vi "AlliGator Select Phasor Plot ROI.vi"(8 "Error In":errorcluster, 11 "ROI Selection Data":cluster{"Action":T1, "ROI ID":i32}) -> (0 "Error Out":errorcluster, 2 "ROI Name":string, 3 "ROI Descriptor":T2 {"Contours"."Type" items=["No Selection", "Point", "Line", "Rectangle", "Oval", "Polygon", "Freehand Region", "Annulus", "Unused2", "Unused3", "Broken Line", "Freehand Line", "Rotated Rectangle"]})   [LabVIEW 2021, in "AlliGator ROIs.lvlib"]
doc: "Handles Phasor Plot image ROI selection."
uses:
  AlliGator ROIs.lvlib
  AlliGator ROI Manager Actions.ctl
  AlliGator Variables List.ctl
  Image/Named ROI Description.ctl
  Variant/Variant to Data/Variant to I32.vi
  <vilib>/Utility/error.llb/Error Cluster From Error Code.vi
  <vilib>/ErrorRing/Error Ring.xnode
  <userlib>/_OpenG.lib/string/string.llb/openg_string.lvlib
  AlliGator Globals, Variables & Constants.lvlib
  Image/Image.lvlib
  Variant/Variant to Data/Variant to Data.lvlib
  Arrays/Arrays.lvlib
panel:
  # "see the AlliGator License on the block diagram (Ctrl+E or Window:Show Block Diagram)"
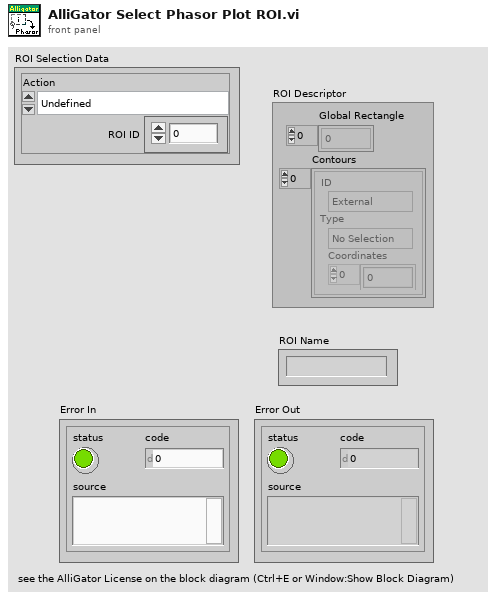
[diagram p1: front panel]
types:
  T1 = typedef "AlliGator ROIs.lvlib/AlliGator ROI Manager Actions.ctl" = enum16{"Undefined", "Delete Current ROI", "Delete All Unselected ROIs", "Delete Multiple ROIs", "Delete All ROIs", "Swap ROIs", "Insert ROI", "Update Current ROI Descriptor", "Rename Current ROI", "Store New ROI", "Store Multiple ROIs", "Select Next ROI", "Select Previous ROI", "Find Selected ROI", "Show All ROIs", "Update ROI Manager Window", "Merge All ROIs", "Unmerge ROI", "Set Selected ROI by ID"}
  T2 = typedef "ROI Descriptor" = cluster{"Global Rectangle":i32[], "Contours":cluster{"ID":enum32{"External", "Internal"}, "Type":u32, "Coordinates":i32[]}[]}
  T3 = typedef "AlliGator Globals, Variables & Constants.lvlib/AlliGator Variables List.ctl" = enum16{"---- GUI ----", "Initialization Status", "State Indicators Refnum", "Original AlliGator Menu Items", "Current Action Loop State", "Script in progress", "Playback", "Loop Playback", "Search ROI Used", "Search ROI", "Decay Graph Max Legend Size", "Intensity Graph Max Legend Size", "Decay Statistics Graph Max Legend Size", "Phasor Graph Max Legend Size", "Phasor Ratio Graph Max Legend Size", "Lifetime Graph Max Legend Size", "---- Files ----", "Export Dataset Frames as Individual Files", "Show Batch Export Help Balloons", "Frames in Dataset", "ptu File Frame Start Indices", "Current Frame in Dataset", "Current Frame Timestamp", "------ Python Plugins ------", "Python Plugins Information", "Python Session", "Valid Python Session?", "---- Source Image ----", "Dataset Loaded", "Dataset Metadata", "Dataset Channel", "Dataset Data Description", "Background Dataset Metadata", "Background Dataset Channel", "Background Dataset Data Description", "Background File Subtraction", "Background File Path", "Background File Pile-up Correction", "Background File Pixel Well Capacity", "Background File Scaling Factor", "Source Image ROIs", "Current Source Image ROI", "Source Image ROI Event Refnum", "X_Source Image Display Range", "X_Source Image Palette Information", "Source Image Palette List", "Source Image Scale", "Current Dataset Load Settings", "Source Image:ROI Overlay Color", "---- Image Profile Window ----", "Image Profile:Overlay ROI in Source Image", "Image Profile Window Event Refnum", "Image Profile:IntensityType", "Image Profile:Intensity Average Type", "Image Profile:Intensity-weighted SDV", "Image Profile:Box Profile Type", "Image Profile Window Open", "Image Profile:Plotted Fit Parameter", "X_Type of Displayed Image", "X_Time Gate Slider", "Dataset Path", "Source Image Overlay to Erase", "Is Displayed Image Accumulated", "White Light Image Modified", "Mask Image Modified", "Macrotime Gate Separation", "------ Phasor Graph -------", "Phasor Graph:Show Line", "---- Phasor Plot ---", "Phasor Plot Parameters Changed", "FLI Dataset Modified since last Phasor Plot Calculation", "Phasor Harmonics Data", "Selected Phasor Harmonics", "Phasor Harmonic Manager Event Refnum", "Phasor Plot ROIs", "Current Phasor Plot ROI", "Phasor Plot ROI Event Refnum", "Phasor Plot Image Reference Points", "Phasor Plot Computed", "Phasor Plot Palette Information", "Phasor Plot Palette List", "Phasor Ratio Palette Information", "Phasor Ratio Palette List", "Phasor Image Scale", "Phasor Plot Image Overlay to Erase", "Phasor Plot Image Elements to Update", "Current Phasor Plot Calculation Parameters", "Current Phasor Calibration Options", "Reset Cumulated Phasor Plot", "Phasor Ratio Reference 1", "Phasor Ratio Lifetime Reference 1", "Phasor Ratio Reference 1 Frequency", "Phasor Ratio Reference 2", "Phasor Ratio Lifetime Reference 2", "Phasor Ratio Reference 2 Frequency", "---- Decay Analysis ----", "Number of Selected Decays to Fit", "LS Fit Results", "LAR Fit Results", "BS Fit Results", "Last Decay Max - Min", "Best Fit Parameters", "Best Fit Parameter Names", "Actual Size X", "Actual Size Y", "Binning X", "Binning Y", "Actual # Gates", "Dataset Number", "Gates to...", "Gates Skipped", "Gates to keep", "Gate Step", "Gate Separation", "Reversed Gates", "Pile-up Correction", "Pixel Well Capacity", "Background Subtracted", "Background Subtraction Method", "Background Definition Range", "Background File (deprecated)", "Number of Dataset Accumulated", "Array of Accumulated Dataset Paths", "Do Averaged Datasets", "Destination File Path", "Process Plot Target", "Use 1/D as Phasor Frequency", "---- Decay Fit Parameter Map -----", "Decay Fit Parameter Map Palette Information", "Decay Fit Parameter Map Palette List", "Local Decay Graph Window Event Refnum", "------- Local Decay Window ---------", "Use normalized IRF for convolution", "----- Miscellaneous ----", "Skippable Dialog Windows Status"}
  T4 = typedef "Image.lvlib/Named ROI Description.ctl" = cluster{"ROI Descriptor":T2, "ROI Name":string, "Overlay Color":u32}
  T5 = typedef "AlliGator ROIs.lvlib/AlliGator Image ROI Event refnum.ctl" = refnum<user-event>
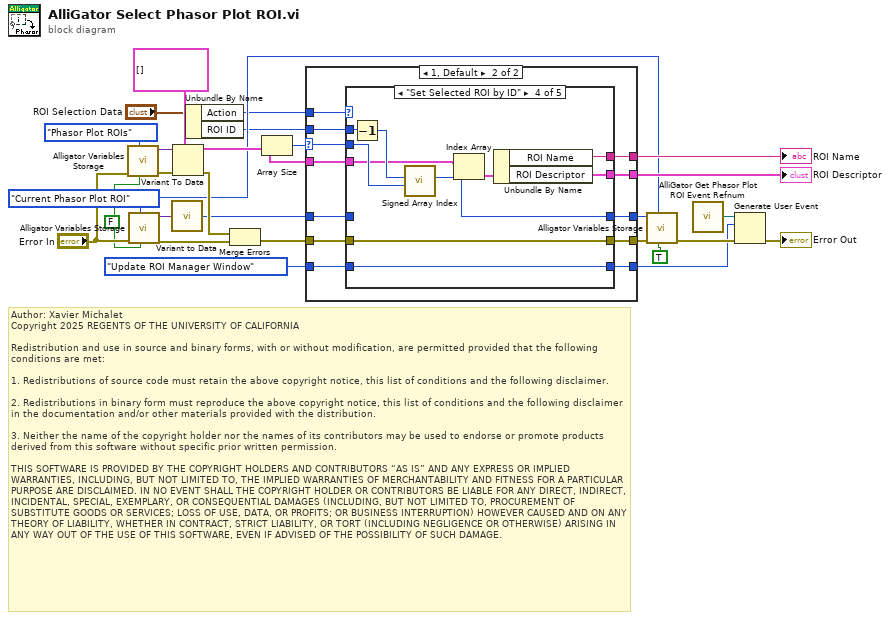
[diagram p0: block diagram]
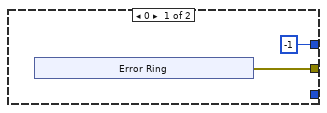
[diagram p2: hidden frame]
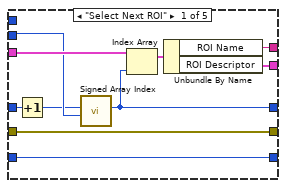
[diagram p3: hidden frame]
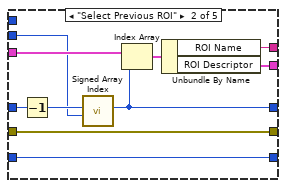
[diagram p4: hidden frame]
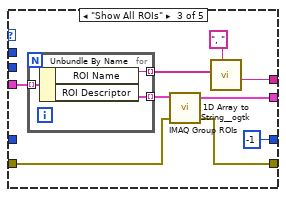
[diagram p5: hidden frame]
diagram:
  w10 = AlliGator_Variables_List."Current Phasor Plot ROI" ("Alligator Variable")
  w17 = FALSE ("Get(F)/Set")
  # "Author: Xavier Michalet\nCopyright 2025 REGENTS OF THE UNIVERSITY OF CALIFORNIA\n\nRedistribution and use in source and binary forms, with or without modification, are permitted provided that the following conditions are met:\n\n1. Redistributions of source code must retain the above copyright notice, this list of conditions and the following disclaimer.\n\n2. Redistributions in binary form must reproduce the above copyright notice, this list of conditions and the following disclaimer in the documentation and/or other materials provided with the distribution.\n\n3. Neither the name of the copyright holder nor the names of its contributors may be used to endorse or promote products derived from this software without specific prior written permission.\n\nTHIS SOFTWARE IS PROVIDED BY THE COPYRIGHT HOLDERS AND CONTRIBUTORS “AS IS” AND ANY EXPRESS OR IMPLIED WARRANTIES, INCLUDING, BUT NOT LIMITED TO, THE IMPLIED WARRANTIES OF MERCHANTABILITY AND FITNESS FOR A PARTICULAR PURPOSE ARE DISCLAIMED. IN NO EVENT SHALL THE COPYRIGHT HOLDER OR CONTRIBUTORS BE LIABLE FOR ANY DIRECT, INDIRECT, INCIDENTAL, SPECIAL, EXEMPLARY, OR CONSEQUENTIAL DAMAGES (INCLUDING, BUT NOT LIMITED TO, PROCUREMENT OF SUBSTITUTE GOODS OR SERVICES; LOSS OF USE, DATA, OR PROFITS; OR BUSINESS INTERRUPTION) HOWEVER CAUSED AND ON ANY THEORY OF LIABILITY, WHETHER IN CONTRACT, STRICT LIABILITY, OR TORT (INCLUDING NEGLIGENCE OR OTHERWISE) ARISING IN ANY WAY OUT OF THE USE OF THIS SOFTWARE, EVEN IF ADVISED OF THE POSSIBILITY OF SUCH DAMAGE."
  n1 = call "Alligator Variables Storage.vi"("Get(F)/Set"=w17, "AlliGator Variable"=AlliGator_Variables_List."Phasor Plot ROIs" ("Alligator Variable"), "Error In"="Error In") -> ("Error Out"=w22:errorcluster, "Data out"=w23:variant)  [unwired: 6 in, 1 out]
  n2 = call "Alligator Variables Storage.vi"("Get(F)/Set"=w17, "AlliGator Variable"=w10, "Error In"="Error In") -> ("Error Out"=w15:errorcluster, "Data out"=w14:variant)  [unwired: 6 in, 1 out]
  n3 = call-poly "Variant to Data.vi"("Variant"=w14) -> ("Value"=w13:i32)  [unwired: 8 in]
  n4 = Variant To Data(error in=w22, type=T4[] [] ("ROIs"), Variant=w23) -> (data=w19:T4[], error out=w20:errorcluster)
  n5 = Unbundle By Name("ROI Selection Data") -> ("Action"=w2:T1, "ROI ID"=w1:i32)
  n6 = Merge Errors(w20, w15) -> (w16:errorcluster)
  n7 = Array Size(array=w19) -> (size(s)=w26:i32)
  n8 = case shown="1, Default" w26 {
    selector: w26 -> [_ w34]
    tunnel: [_ w45] -> w27
    tunnel: [-1 w44] -> w12
    tunnel: w13 -> [_ w43]
    tunnel: w2 -> [_ w42]
    tunnel: w19 -> [_ w41]
    tunnel: w16 -> [_ w40]
    tunnel: [w28 w39] -> w9
    tunnel: [_ w38] -> w25
    tunnel: AlliGator_ROI_Manager_Actions."Update ROI Manager Window" ("event data") -> [_ w37]
    tunnel: [_ w36] -> w3
    tunnel: w1 -> [_ w35]
    frame 0 {
      n9 = xnode "Error Ring"() -> ("error out"=w28:errorcluster)
    }
    frame 1, Default {
      n10 = case shown="\"Set Selected ROI by ID\"" w42 {
        tunnel: w41 -> [w50 w65 w71 w81 _]
        tunnel: w43 -> [w48 w63 _ _ w88]
        tunnel: [w47 w56 -1 ("Value") w80 w88] -> w44
        tunnel: [w53 w61 w74 w83 _] -> w45
        tunnel: w34 -> [w49 w57 _ w85 _]
        tunnel: w40 -> [w54 w62 w73 w78 w89]
        tunnel: [w54 w62 w72 w78 w89] -> w39
        tunnel: [w52 w60 w68 w84 _] -> w38
        tunnel: w37 -> [w51 w59 _ w79 _]
        tunnel: [w51 w59 _ w79 _] -> w36
        tunnel: w35 -> [_ _ _ w86 _]
        frame "Select Next ROI" {
          n11 = Increment(x=w48) -> (x+1=w46:i32)
          n12 = call "Signed Array Index.vi"("Array Size"=w49, "Array Index in"=w46) -> ("Array Index out"=w47:i32)  [unwired: 9 in]
          n13 = Index Array(array=w50, index=w47) -> (element=w55:T4)
          n14 = Unbundle By Name(w55) -> ("ROI Name"=w52:string, "ROI Descriptor"=w53:T2)
        }
        frame "Select Previous ROI" {
          n15 = Decrement(x=w63) -> (x-1=w58:i32)
          n16 = call "Signed Array Index.vi"("Array Size"=w57, "Array Index in"=w58) -> ("Array Index out"=w56:i32)  [unwired: 9 in]
          n17 = Index Array(array=w65, index=w56) -> (element=w64:T4)
          n18 = Unbundle By Name(w64) -> ("ROI Name"=w60:string, "ROI Descriptor"=w61:T2)
        }
        frame "Show All ROIs" {
          n19 = for {
            tunnel: w71 -> [w77] mode=indexing
            tunnel: [w76] -> w70 mode=indexing
            tunnel: [w75] -> w69 mode=indexing
            n20 = Unbundle By Name(w77) -> ("ROI Name"=w75:string, "ROI Descriptor"=w76:T2)
          }
          n21 = call "IMAQ Group ROIs"("error in (no error)"=w73, "ROI Descriptors"=w70) -> ("error out"=w72:errorcluster, "ROI Descriptor out"=w74:T2)  [unwired: 2 in]
          n22 = call <userlib>:"1D Array to String__ogtk.vi"("delimiter (Tab)"=", ", "Array of Strings"=w69) -> ("delimited string"=w68:string)  [unwired: 9 in]
        }
        frame "Set Selected ROI by ID" {
          n23 = Decrement(x=w86) -> (x-1=w87:i32)
          n24 = call "Signed Array Index.vi"("Array Size"=w85, "Array Index in"=w87) -> ("Array Index out"=w80:i32)  [unwired: 9 in]
          n25 = Index Array(array=w81, index=w80) -> (element=w82:T4)
          n26 = Unbundle By Name(w82) -> ("ROI Name"=w84:string, "ROI Descriptor"=w83:T2)
        }
        frame Default {
        }
      }
    }
  }
  "ROI Descriptor" <- w27
  "ROI Name" <- w25
  n27 = call "Alligator Variables Storage.vi"("Get(F)/Set"=TRUE, "AlliGator Variable"=w10, "Error In"=w9, "Data in"=w12) -> ("Error Out"=w6:errorcluster)  [unwired: 5 in, 2 out]
  n28 = call "AlliGator Get Phasor Plot ROI Event Refnum.vi"() -> ("Phasor Plot ROI Event Refnum"=w7:T5)
  n29 = Generate User Event(user event=w7, event data cluster=w3, error in=w6) -> (error out=→"Error Out":errorcluster)  [unwired: 1 in, 1 out]
